vi "Append Dictionary (Loop).vi"(8 "error in (no error)":errorcluster, 10 "key-values":T1[](array[typedef]), 11 "Control Experiment":refnum<class "Control Experiment.lvclass">) -> (0 "error out":errorcluster, 3 "Control Experiment out":refnum<class "Control Experiment.lvclass">)   [LabVIEW 2019, in "Control Experiment.lvclass"]
uses:
  Control Experiment.lvclass
  <userlib>/LevyLab/LV-Data/LV-Data/Typedefs/Dictionary--cluster.ctl
  <userlib>/LevyLab/LV-Data/LV-Data/LV-Data.lvclass
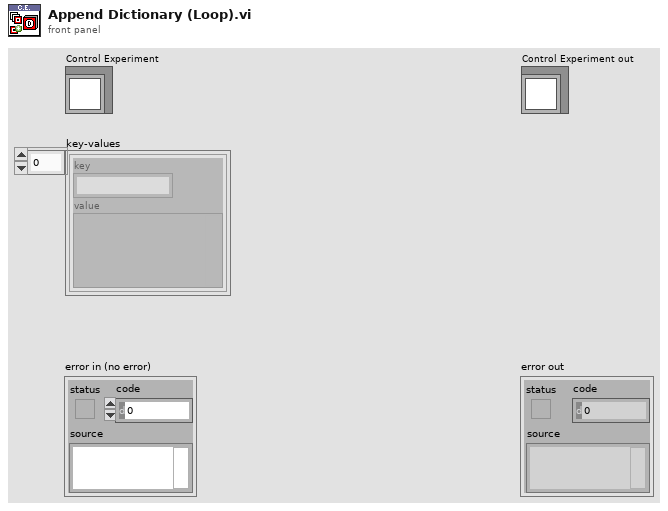
[diagram p1: front panel]
types:
  T1 = typedef "LV-Data.lvclass/Dictionary--cluster.ctl" = cluster{"key":string, "value":variant}
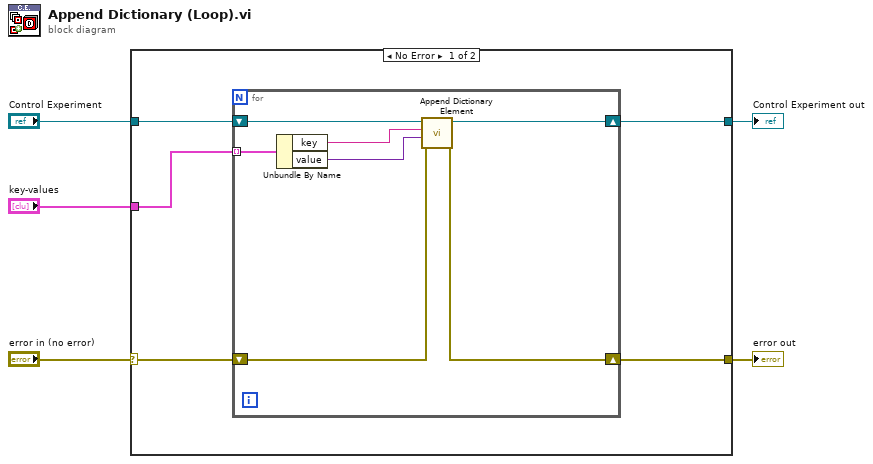
[diagram p0: block diagram]
diagram:
  n1 = case shown="No Error" "error in (no error)" {
    selector: "error in (no error)" -> [w7 w18]
    tunnel: [w6 w18] -> w4
    tunnel: [w8 w19] -> w2
    tunnel: "Control Experiment" -> [w9 w19]
    tunnel: "key-values" -> [w10 _]
    frame No Error {
      n2 = for {
        tunnel: w10 -> [w17] mode=indexing
        shift-right: [w15] -> w8
        shift-left: w9 -> [w16]
        shift-right: [w11] -> w6
        shift-left: w7 -> [w12]
        n3 = Unbundle By Name(w17) -> ("key"=w14:string, "value"=w13:variant)
        n4 = call "Append Dictionary Element.vi"("error in (no error)"=w12, "value"=w13, "key"=w14, "Control Experiment"=w16) -> ("error out"=w11:errorcluster, "Control Experiment out"=w15:refnum<class "Control Experiment.lvclass">)  [unwired: 6 in]
      }
    }
    frame Error {
    }
  }
  "error out" <- w4
  "Control Experiment out" <- w2
